vi "Get 1D Pixel Array.vi"(11 "image data":T1) -> (3 "1D Pixel Array":u32[](array[numeric]))   [LabVIEW 2014, in "Image Comparison.lvclass"]
uses:
  Image Comparison.lvclass
  <vilib>/picture/picture.llb/imagedata.ctl
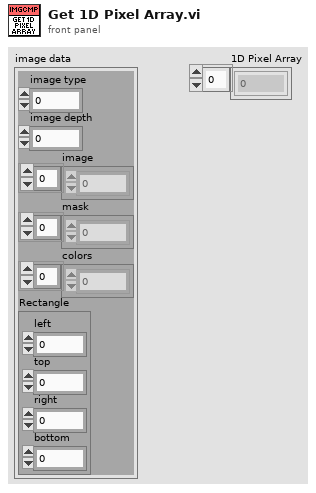
[diagram p1: front panel]
types:
  T1 = typedef "imagedata.ctl" = cluster{"image type":i32, "image depth":i32, "image":u8[], "mask":u8[], "colors":u32[], "Rectangle":cluster{"left":i16, "top":i16, "right":i16, "bottom":i16}}
  T2 = cluster{"left":i16, "top":i16, "right":i16, "bottom":i16}
  T3 = cluster{"left":i32, "top":i32, "right":i32, "bottom":i32}
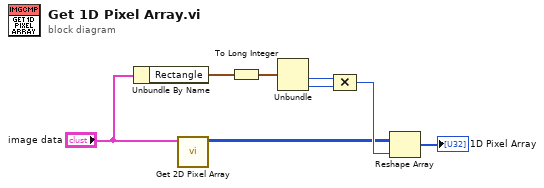
[diagram p0: block diagram]
diagram:
  n1 = Unbundle By Name("image data") -> ("Rectangle"=w2:T2)
  n2 = call "Get 2D Pixel Array.vi"("image data"="image data") -> ("2D Pixel Array"=w5:u32[][])  [unwired: 10 in]
  n3 = To Long Integer(number=w2) -> (32bit integer=w7:T3)
  n4 = Unbundle(w7) -> ("right"=w3:i32, "bottom"=w4:i32)  [unwired: 2 out]
  n5 = Compound Arithmetic op=MULTIPLY(w3, w4) -> (w6:i32)
  n6 = Reshape Array(w5, w6) -> (→"1D Pixel Array":u32[])
